vi "URL_Parameters_Update.vi"(0 "Google Maps Resource In":T1, 7 "URL Parameter":cluster{"Key":string, "Value":string}) -> (4 "Google Maps Resource Out":T1)   [LabVIEW 2020]
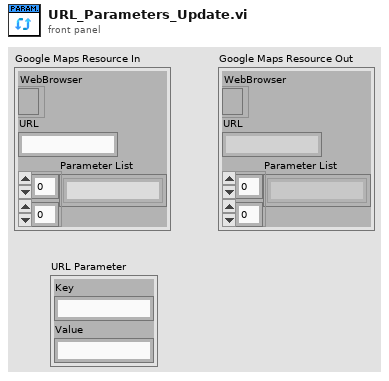
[diagram p1: front panel]
types:
  T1 = cluster{"WebBrowser":refnum<k7>, "URL":string, "Parameter List":string[][]}
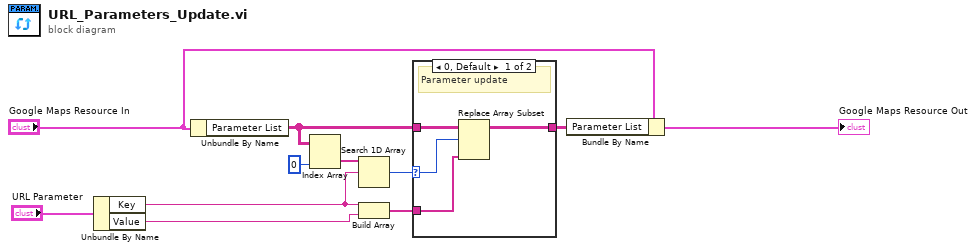
[diagram p0: block diagram]
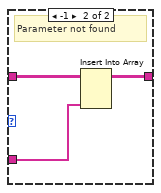
[diagram p2: hidden frame]
diagram:
  n1 = Unbundle By Name("URL Parameter") -> ("Key"=w1:string, "Value"=w2:string)
  n2 = Unbundle By Name("Google Maps Resource In") -> ("Parameter List"=w7:string[][])
  n3 = Index Array(array=w7, index (col)=0 ("disabled index (col)")) -> (element=w5:string[])  [unwired: 1 in]
  n4 = Search 1D Array(1D array=w5, element=w1) -> (index of element=w6:i32)  [unwired: 1 in]
  n5 = Build Array(w1, w2) -> (w8:string[])
  n6 = case shown="0, Default" w6 {
    selector: w6 -> [w12 _]
    tunnel: w7 -> [w15 w18]
    tunnel: [w13 w17] -> w9
    tunnel: w8 -> [w14 w16]
    frame 0, Default {
      # "Parameter update"
      n7 = Replace Array Subset(array=w15, new element=w14, index (row)=w12) -> (w13:string[][])  [unwired: 1 in]
    }
    frame -1 {
      # "Parameter not found"
      n8 = Insert Into Array(array=w18, new element=w16) -> (w17:string[][])  [unwired: 2 in]
    }
  }
  n9 = Bundle By Name(cluster="Google Maps Resource In", "Parameter List"=w9) -> (→"Google Maps Resource Out":T1)
